vi "8bit truecolor.vi"(0 "8bit truecolor":u8) -> (2 "red":u8, 3 "green":u8, 4 "blue":u8)   [LabVIEW 2009]
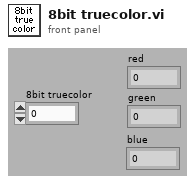
[diagram p1: front panel]
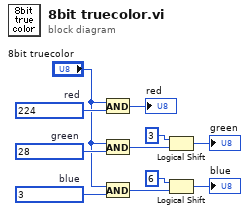
[diagram p0: block diagram]
diagram:
  w7 = u8 3  # blue
  w9 = u8 28  # green
  w11 = u8 224  # red
  n1 = And(x="8bit truecolor", y=w11) -> (x .and. y?=→"red":u8)
  n2 = And(x="8bit truecolor", y=w9) -> (x .and. y?=w6:u8)
  n3 = And(x="8bit truecolor", y=w7) -> (x .and. y?=w3:u8)
  n4 = Logical Shift(y=i8 3, x=w6) -> (x << y=→"green":u8)
  n5 = Logical Shift(y=i8 6, x=w3) -> (x << y=→"blue":u8)
